vi "Make.vi"(8 "error in (no error)":errorcluster, 9 "Item Refnum":refnum<vi>, 10 "Target":refnum<vi>, 11 "Message Scripter":refnum<class "Message Scripter.lvclass">) -> (0 "error out":errorcluster, 3 "Message Scripter out":refnum<class "Message Scripter.lvclass">)   [LabVIEW 2020, in "Message Maker.lvlib" / "Message Scripter.lvclass"]
uses:
  Message Scripter.lvclass
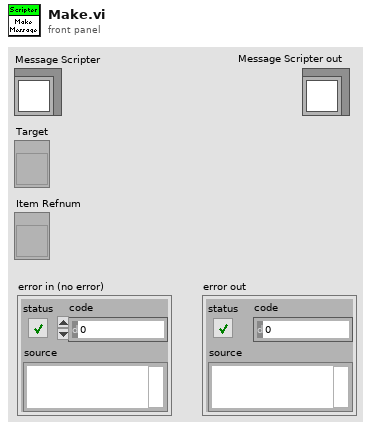
[diagram p1: front panel]
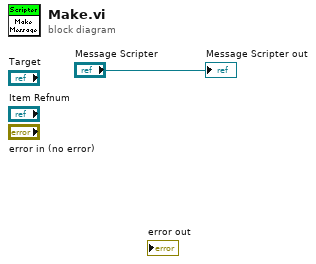
[diagram p0: block diagram]
diagram:
  "Message Scripter out" <- "Message Scripter"
